vi "uncluster.vi"() -> ()   [LabVIEW 2021]
panel:
  out "Boolean 8":bool
  out "Boolean 7":bool
  out "Boolean 6":bool
  out "Boolean 5":bool
  out "Boolean 4":bool
  out "Boolean 3":bool
  out "Boolean 2":bool
  out "Boolean":bool
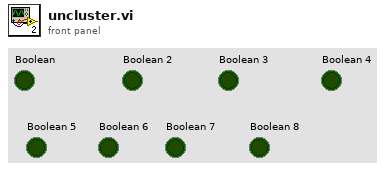
[diagram p1: front panel]
types:
  T1 = cluster{bool, bool, bool, bool, bool, bool, bool, bool}
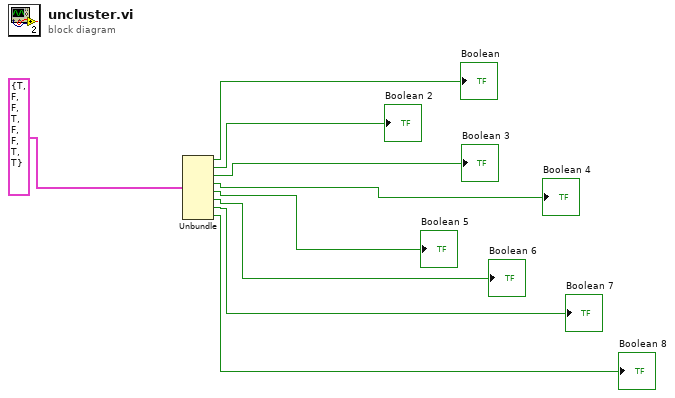
[diagram p0: block diagram]
diagram:
  n1 = Unbundle(T1 {TRUE, FALSE, FALSE, TRUE, FALSE, FALSE, TRUE, TRUE}) -> (→"Boolean":bool, →"Boolean 2":bool, →"Boolean 3":bool, →"Boolean 4":bool, →"Boolean 5":bool, →"Boolean 6":bool, →"Boolean 7":bool, →"Boolean 8":bool)
